vi "DNS显示.vi"(11 "DNS数组":u8[](array[numeric])) -> (3 "输出显示":string)   [LabVIEW 2015]
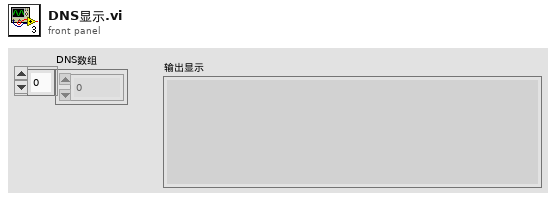
[diagram p1: front panel]
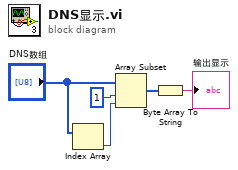
[diagram p0: block diagram]
diagram:
  n1 = Index Array(array="DNS数组") -> (element=w3:u8)  [unwired: 1 in]
  n2 = Array Subset(array="DNS数组", index=1 ("索引"), length=w3) -> (w2:u8[])
  n3 = Byte Array To String(unsigned byte array=w2) -> (string=→"输出显示":string)
